vi "Database Change Manager UI.vi"(8 "error in (no error)":errorcluster, 10 "Old Cluster":refnum<k21>, 11 "VS Existing Frames":T1 {"Incoming"."Node Ref" format="%.0x"; "Outgoing"."Node Ref" format="%.0x"}) -> (0 "error out":errorcluster, 2 "Cancel Out":bool, 3 "Change":T5 {"Outgoing"."Frames to Update"."Node Ref" format="%.0x"; "Outgoing"."Frames to Delete" format="%.0x"; "Incoming"."Frames to Update"."Node Ref" format="%.0x"; "Incoming"."Frames to Delete" format="%.0x"})   [LabVIEW 2025, in "Protection and Counter Addon System Explorer.lvlib"]
uses:
  Protection and Counter Addon System Explorer.lvlib
  Types/CAN Update Results.ctl
  Types/VS Update List.ctl
  <vilib>/NI VeriStand/Custom Device API/Custom Device Item Ref.ctl
  Types/Base Frame Info_NoVS.ctl
  Types/Signal Attributes.ctl
  Types/CAN Filter Type.ctl
  Types/CAN Frame Update Results.ctl
  Types/Database Changes VS Existing Frames.ctl
  Types/Base Frame Info.ctl
  <vilib>/Utility/cursorutil.llb/Set Cursor (Icon Pict).vi
  <resource>/objmgr/xnet.rc
  <vilib>/NI VeriStand/Custom Device API/Custom Device API.lvlib
panel:
  in  "New Cluster":u16(ring)
  in  "New Database":refnum<k21>
  in  "Export":bool
  in  "Cancel":bool
  in  "Update":bool
  in  "Tree":string(tree)
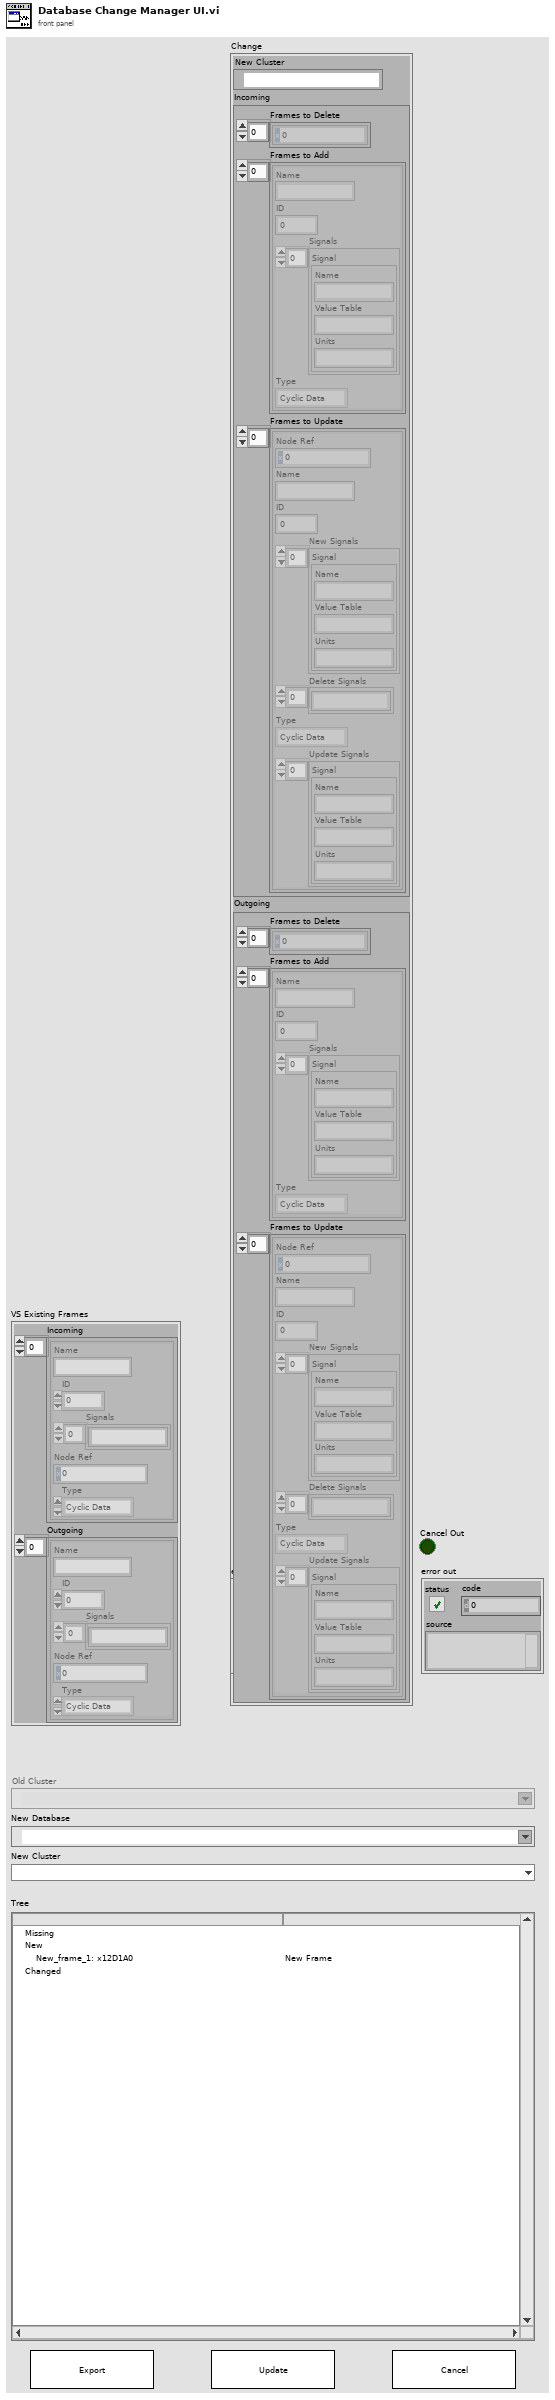
[diagram p1: front panel]
types:
  T1 = typedef "Protection and Counter Addon System Explorer.lvlib/Database Changes VS Existing Frames.ctl" = cluster{"Incoming":T2[], "Outgoing":T2[]}
  T2 = typedef "Protection and Counter Addon System Explorer.lvlib/Base Frame Info.ctl" = cluster{"Name":string, "ID":u32, "Signals":string[], "Node Ref":T3, "Type":T4}
  T3 = typedef "Custom Device API.lvlib/Custom Device Item Ref.ctl" = u64
  T4 = typedef "Protection and Counter Addon System Explorer.lvlib/CAN Filter Type.ctl" = enum16{"Cyclic Data", "Event Data", "Cyclic/Event", "All"}
  T5 = typedef "Protection and Counter Addon System Explorer.lvlib/CAN Update Results.ctl" = cluster{"New Cluster":refnum<k21>, "Incoming":T6, "Outgoing":T6}
  T6 = typedef "Protection and Counter Addon System Explorer.lvlib/VS Update List.ctl" = cluster{"Frames to Delete":T3[], "Frames to Add":T7[], "Frames to Update":T9[]}
  T7 = typedef "Protection and Counter Addon System Explorer.lvlib/Base Frame Info_NoVS.ctl" = cluster{"Name":string, "ID":u32, "Signals":T8[], "Type":T4}
  T8 = typedef "Protection and Counter Addon System Explorer.lvlib/Signal Attributes.ctl" = cluster{"Name":string, "Value Table":string, "Units":string}
  T9 = typedef "Protection and Counter Addon System Explorer.lvlib/CAN Frame Update Results.ctl" = cluster{"Node Ref":T3, "Name":string, "ID":u32, "New Signals":T8[], "Delete Signals":string[], "Type":T4, "Update Signals":T8[]}
  T10 = enum8{"Enabled", "Disabled", "Disabled and Grayed Out"}
  T11 = typedef "Protection and Counter Addon System Explorer.lvlib/Filtered XNET Changes.ctl" = cluster{"Incoming":T12, "Outgoing":T12}
  T12 = typedef "Protection and Counter Addon System Explorer.lvlib/Database Changes.ctl" = cluster{"New":T7[], "Missing":T2[], "Changed":T13[]}
  T13 = typedef "Protection and Counter Addon System Explorer.lvlib/Related CAN Frames.ctl" = cluster{"Old":T2, "Change":T14}
  T14 = typedef "Protection and Counter Addon System Explorer.lvlib/Related CAN Frames No VS.ctl" = cluster{"New":T7, "Old":T7}
  T15 = typedef "LVPoint32TypeDef.ctl" = cluster{"Horizontal":i32, "Vertical":i32}
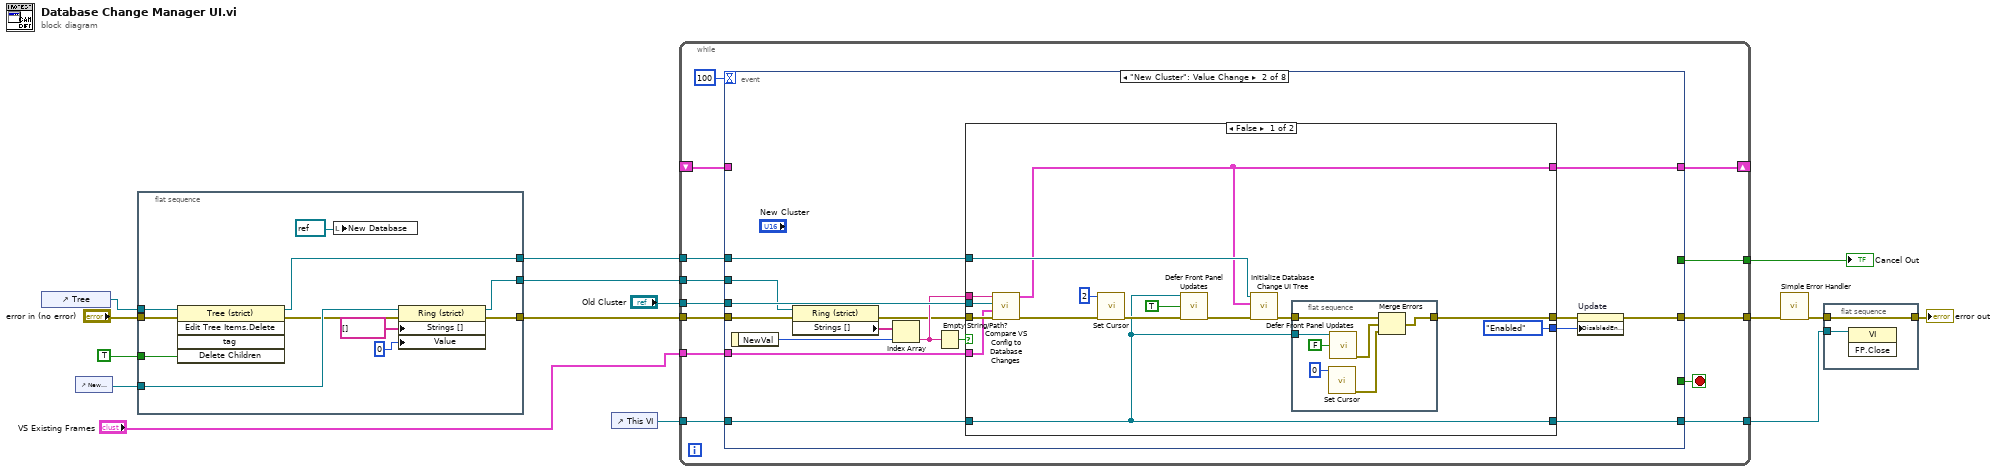
[diagram p0: block diagram]
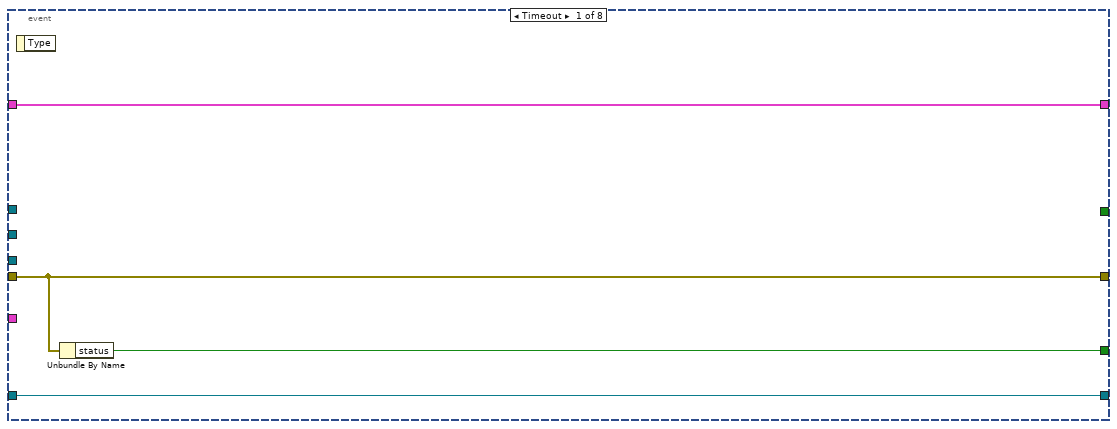
[diagram p2: hidden frame]
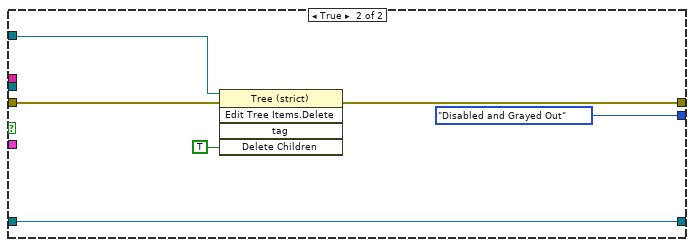
[diagram p3: hidden frame]
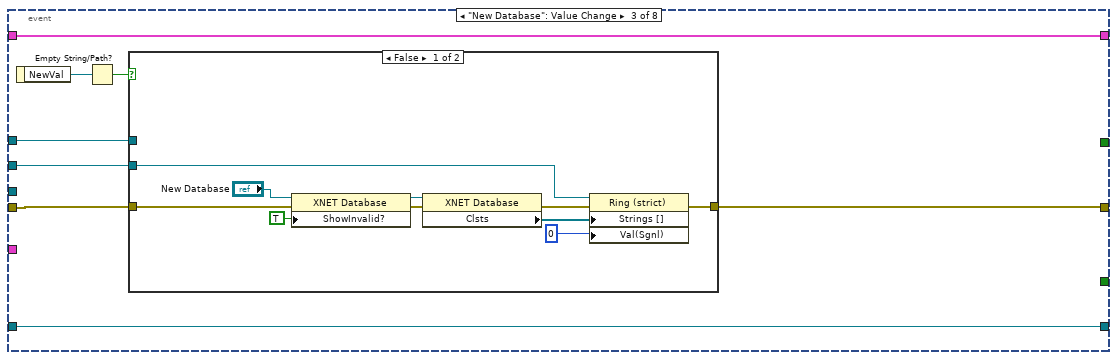
[diagram p4: hidden frame]
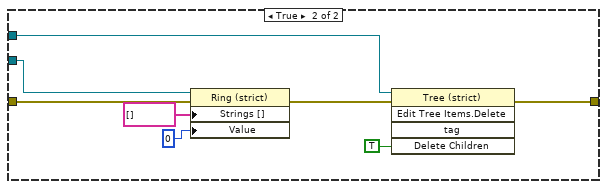
[diagram p5: hidden frame]
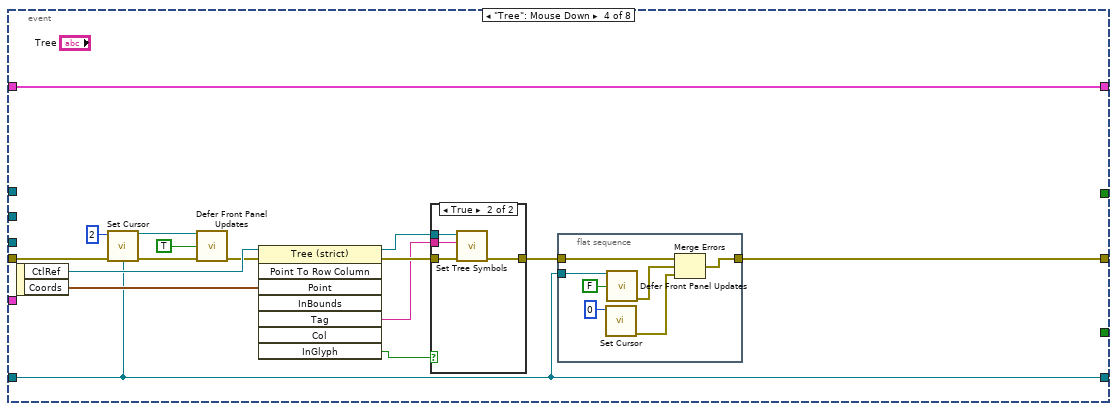
[diagram p6: hidden frame]
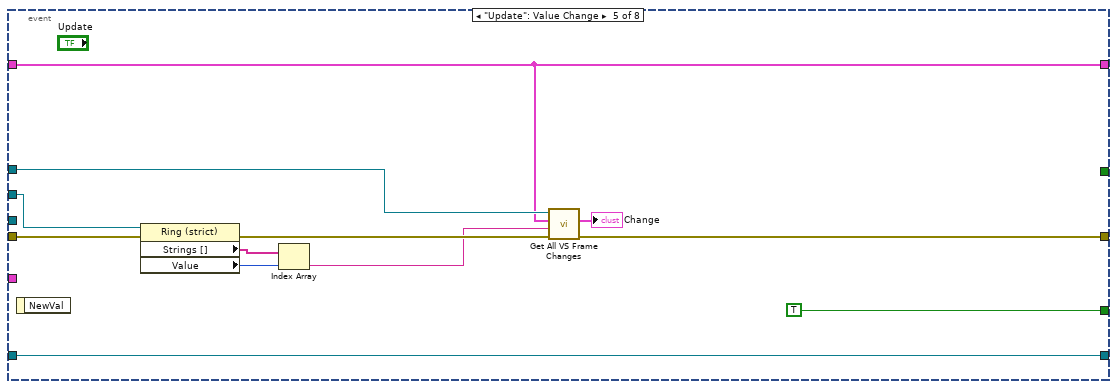
[diagram p8: hidden frame]
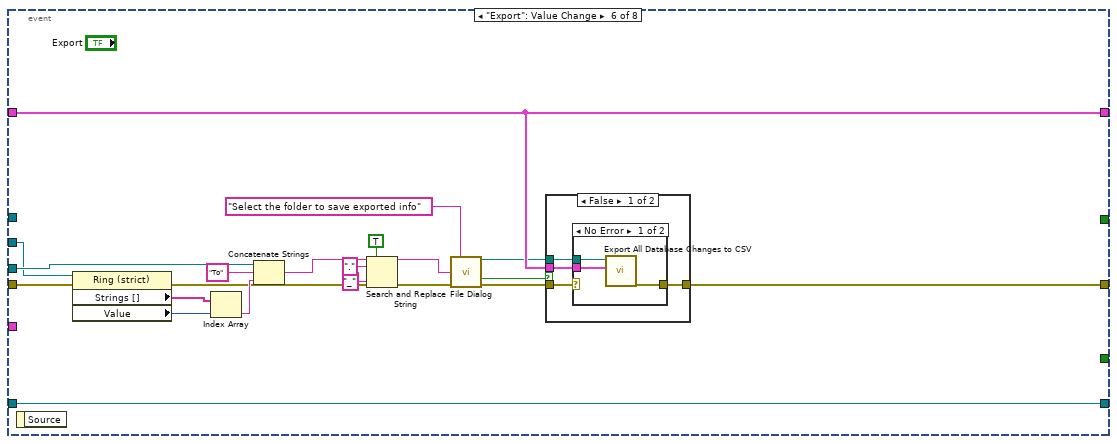
[diagram p9: hidden frame]
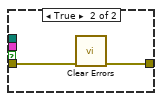
[diagram p11: hidden frame]
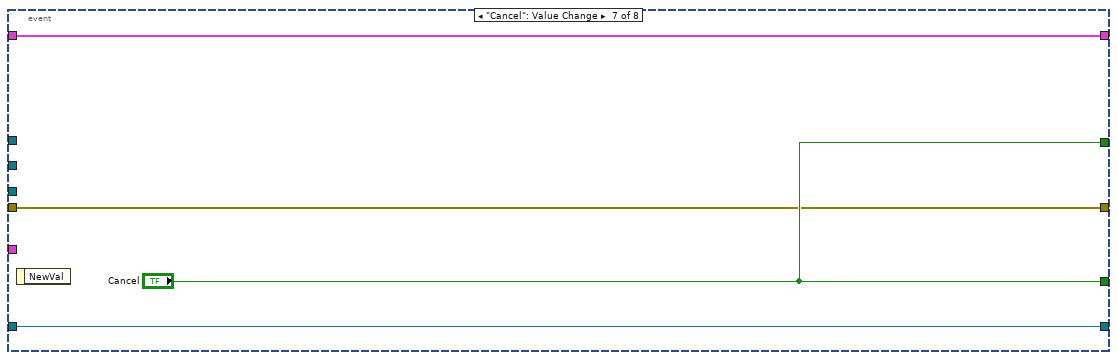
[diagram p12: hidden frame]
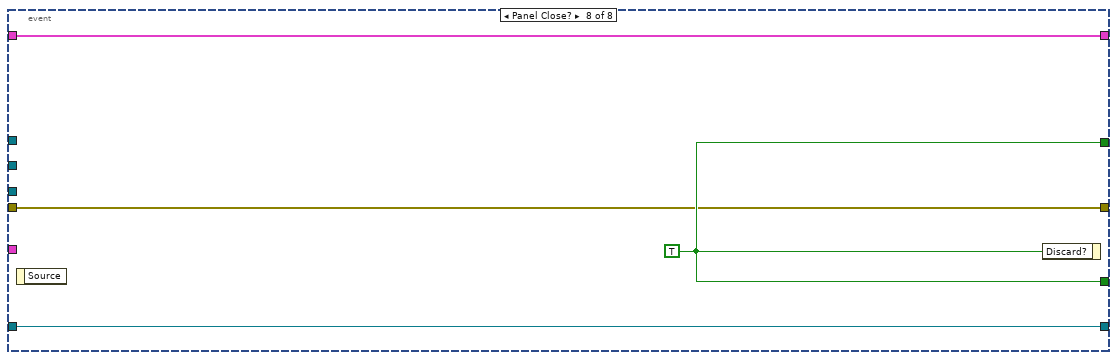
[diagram p13: hidden frame]
diagram:
  n1 = control-ref of="Tree"() -> (w7:refnum<vi>)
  n2 = control-ref of="New Cluster"() -> (w3:refnum<vi>)
  n3 = flat-sequence {
    tunnel: TRUE ("Delete Children?") -> [w26]
    tunnel: w7 -> [w25]
    tunnel: [w24] -> w6
    tunnel: "error in (no error)" -> [w23]
    tunnel: [w18] -> w4
    tunnel: w3 -> [w22]
    tunnel: [w17] -> w2
    frame #0 {
      n4 = invoke on="Invoke Node" class="Tree (strict)" method="Edit Tree Items.Delete"(reference=w25, error in=w23, "Delete Children"=w26) -> (reference out=w24:refnum<vi>, error out=w19:errorcluster)  [unwired: 2 in, 3 out]
      n5 = local write "New Database"(refnum<k21> refnum ("New Database")) -> ()
      n6 = property on="Property Node" class="Ring (strict)"(reference=w22, error in=w19, "Strings []"=string[] [], "Value"=u16 0) -> (reference out=w17:refnum<vi>, error out=w18:errorcluster)
    }
  }
  n7 = control-ref of="This VI"() -> (w9:refnum<vi>)
  n8 = while {
    tunnel: [w38] -> w14
    tunnel: [w37] -> w13
    tunnel: [w36] -> w12
    tunnel: "Old Cluster" -> [w34]
    tunnel: w6 -> [w33]
    tunnel: w9 -> [w32]
    tunnel: w4 -> [w31]
    shift-right: [w30] -> _
    shift-left: _ -> [w29]
    tunnel: "VS Existing Frames" -> [w28]
    tunnel: w2 -> [w27]
    stop <- w39 stop-if-true
    n9 = event shown="[1] \"New Cluster\": Value Change" {
      selector: _ -> [_ _ _ _ _ _ _ _]
      dyn-events: _ -> [_ _ _ _ _ _ _ _]
      timeout: 100 -> [_ _ _ _ _ _ _ _]
      tunnel: [w43 _ _ _ TRUE ("status") _ "Cancel" w191] -> w39
      tunnel: [w42 w52 w90 w120 w151 w153 w186 w190] -> w38
      tunnel: [w41 w55 w89 w116 w150 w173 w185 w189] -> w37
      tunnel: [_ _ _ _ _ _ "Cancel" w191] -> w36
      tunnel: w34 -> [_ w59 _ _ _ w168 _ _]
      tunnel: w33 -> [_ w58 w88 _ w149 _ _ _]
      tunnel: w32 -> [w41 w57 w89 w116 w150 w173 w185 w189]
      tunnel: w31 -> [w42 w45 w92 w115 w144 w163 w186 w190]
      tunnel: [w40 w56 w95 w114 w148 w172 w184 w188] -> w30
      tunnel: w29 -> [w40 _ w95 w114 w148 w172 w184 w188]
      tunnel: w28 -> [_ w50 _ _ _ _ _ _]
      tunnel: w27 -> [_ w44 w91 _ w146 w164 _ _]
      event Timeout {
        n10 = event-data() -> ()  [unwired: 1 in, 1 out]
        n11 = Unbundle By Name(w42) -> ("status"=w43:bool)
      }
      event "New Cluster": Value Change {
        n12 = event-data() -> ("NewVal"=w48:u16)  [unwired: 1 in]
        n13 = property class="Ring (strict)"(reference=w44, error in=w45) -> (error out=w46:errorcluster, "Strings []"=w49:string[])  [unwired: 1 out]
        n14 = Index Array(array=w49, index=w48) -> (element=w47:string)
        n15 = Empty String/Path?(string/path=w47) -> (empty?=w54:bool)
        n16 = case shown="False" w54 {
          tunnel: w59 -> [w71 _]
          tunnel: w47 -> [w70 _]
          tunnel: w58 -> [w69 w82]
          tunnel: w46 -> [w66 w83]
          tunnel: w57 -> [w63 w87]
          tunnel: [w64 w84] -> w53
          tunnel: [w60 _] -> w56
          tunnel: [w63 w87] -> w55
          tunnel: [T10."Enabled" ("Disabled") T10."Disabled and Grayed Out" ("Disabled")] -> w51
          tunnel: w50 -> [w61 _]
          frame False {
            n17 = call "Compare VS Config to Database Changes.vi"("error in (no error)"=w66, "VS Existing Frames"=w61, "Old Cluster"=w71, "New Cluster"=w70) -> ("error out"=w65:errorcluster, "VS Filtered Change List"=w60:T11)  [unwired: 6 in]
            n18 = call-poly <vilib>:"Set Cursor.vi"("error in (no error)"=w65, "icon"=u16 2) -> ("error out"=w72:errorcluster)  [unwired: 8 in, 1 out]
            n19 = call "Defer Front Panel Updates.vi"("This VI"=w63, "Defer Panel Updates"=TRUE, "error in (no error)"=w72) -> ("error out"=w73:errorcluster)  [unwired: 12 in]
            n20 = call "Initialize Database Change UI Tree.vi"("error in (no error)"=w73, "VS Filtered Change List"=w60, "TreeControl in"=w69) -> ("error out"=w74:errorcluster)  [unwired: 7 in, 1 out]
            n21 = flat-sequence {
              tunnel: [w80] -> w64
              tunnel: w74 -> [w79]
              tunnel: w63 -> [w77]
              frame #0 {
                n22 = call-poly <vilib>:"Set Cursor.vi"("icon"=u16 0) -> ("error out"=w75:errorcluster)  [unwired: 9 in, 1 out]
                n23 = call "Defer Front Panel Updates.vi"("This VI"=w77, "Defer Panel Updates"=FALSE) -> ("error out"=w78:errorcluster)  [unwired: 13 in]
                n24 = Merge Errors(w79, w78, w75) -> (w80:errorcluster)
              }
            }
          }
          frame True {
            n25 = invoke on="Invoke Node" class="Tree (strict)" method="Edit Tree Items.Delete"(reference=w82, error in=w83, "Delete Children"=TRUE ("Delete Children?")) -> (error out=w84:errorcluster)  [unwired: 2 in, 4 out]
          }
        }
        n26 = property on="Update" class="Bool"(error in=w53, "DisabledEnum"=w51) -> (error out=w52:errorcluster)  [unwired: 1 in, 1 out]
      }
      event "New Database": Value Change {
        n27 = event-data() -> ("NewVal"=w94:refnum<k21>)  [unwired: 1 in]
        n28 = Empty String/Path?(string/path=w94) -> (empty?=w93:bool)
        n29 = case shown="False" w93 {
          tunnel: w92 -> [w100 w106]
          tunnel: w91 -> [w98 w108]
          tunnel: [w96 w111] -> w90
          tunnel: w88 -> [_ w113]
          frame False {
            n30 = property class="XNET Database"(reference="New Database", error in=w100, "ShowInvalid?"=TRUE ("Show Invalid From Open?")) -> (reference out=w105:refnum<k21>, error out=w104:errorcluster)
            n31 = property class="XNET Database"(reference=w105, error in=w104) -> (error out=w97:errorcluster, "Clsts"=w101:refnum<k21>[])  [unwired: 1 out]
            n32 = property on="Property Node" class="Ring (strict)"(reference=w98, error in=w97, "Strings []"=w101, "Val(Sgnl)"=u16 0 ("Value (Signaling)")) -> (error out=w96:errorcluster)  [unwired: 1 out]
          }
          frame True {
            n33 = property on="Property Node" class="Ring (strict)"(reference=w108, error in=w106, "Strings []"=string[] [], "Value"=u16 0) -> (error out=w107:errorcluster)  [unwired: 1 out]
            n34 = invoke on="Invoke Node" class="Tree (strict)" method="Edit Tree Items.Delete"(reference=w113, error in=w107, "Delete Children"=TRUE ("Delete Children?")) -> (error out=w111:errorcluster)  [unwired: 2 in, 4 out]
          }
        }
      }
      event "Tree": Mouse Down {
        n35 = event-data() -> ("CtlRef"=w127:refnum<vi>, "Coords"=w128:T15)  [unwired: 1 in]
        n36 = call-poly <vilib>:"Set Cursor.vi"("error in (no error)"=w115, "icon"=u16 2) -> ("error out"=w118:errorcluster)  [unwired: 8 in, 1 out]
        n37 = call "Defer Front Panel Updates.vi"("This VI"=w116, "Defer Panel Updates"=TRUE, "error in (no error)"=w118) -> ("error out"=w117:errorcluster)  [unwired: 12 in]
        n38 = invoke on="Invoke Node" class="Tree (strict)" method="Point To Row Column"(reference=w127, error in=w117, "Point"=w128) -> (reference out=w125:refnum<vi>, error out=w126:errorcluster, "Tag"=w124:string, "InGlyph"=w123:bool)  [unwired: 5 in, 4 out]
        n39 = case shown="True" w123 {
          tunnel: w126 -> [w136 w140]
          tunnel: w125 -> [_ w139]
          tunnel: w124 -> [_ w138]
          tunnel: [w136 w137] -> w121
          frame False {
          }
          frame True {
            n40 = call "Set Tree Symbols.vi"("error in"=w140, "Tag"=w138, "CtlRef"=w139) -> ("error out"=w137:errorcluster)  [unwired: 8 in]
          }
        }
        n41 = flat-sequence {
          tunnel: [w132] -> w120
          tunnel: w121 -> [w133]
          tunnel: w116 -> [w129]
          frame #0 {
            n42 = call-poly <vilib>:"Set Cursor.vi"("icon"=u16 0) -> ("error out"=w134:errorcluster)  [unwired: 9 in, 1 out]
            n43 = call "Defer Front Panel Updates.vi"("This VI"=w129, "Defer Panel Updates"=FALSE) -> ("error out"=w130:errorcluster)  [unwired: 13 in]
            n44 = Merge Errors(w133, w130, w134) -> (w132:errorcluster)
          }
        }
      }
      event "Update": Value Change {
        n45 = event-data() -> ()  [unwired: 1 in, 1 out]
        n46 = property on="Property Node" class="Ring (strict)"(reference=w146, error in=w144) -> (error out=w145:errorcluster, "Strings []"=w143:string[], "Value"=w142:u16)  [unwired: 1 out]
        n47 = Index Array(array=w143, index=w142) -> (element=w141:string)
        n48 = call "Get All VS Frame Changes.vi"("error in (no error)"=w145, "New Cluster"=w141, "VS Filtered Change List"=w148, "TreeControl in"=w149) -> ("error out"=w151:errorcluster, "Change"=→"Change":T5)  [unwired: 5 in, 1 out]
      }
      event "Export": Value Change {
        n49 = event-data() -> ()  [unwired: 1 in, 1 out]
        n50 = property on="Property Node" class="Ring (strict)"(reference=w164, error in=w163) -> (error out=w159:errorcluster, "Strings []"=w162:string[], "Value"=w165:u16)  [unwired: 1 out]
        n51 = Index Array(array=w162, index=w165) -> (element=w161:string)
        n52 = Concatenate Strings(w168, "To" ("string"), w161) -> (w157:string)
        n53 = Search and Replace String(replace all?=TRUE ("replace all? (F)"), input string=w157, search string=".", replace string="_" ("replace string (\"\")"), error in=w159) -> (result string=w160:string, error out=w158:errorcluster)  [unwired: 3 in, 2 out]
        n54 = call "File Dialog"("prompt"="Select the folder to save exported info", "default name"=w160, "error in"=w158) -> ("selected path"=w171:path, "cancelled"=w170:bool, "error out"=w169:errorcluster)  [unwired: 9 in, 1 out]
        n55 = case shown="False" w170 {
          tunnel: w172 -> [w177 _]
          tunnel: w171 -> [w176 _]
          tunnel: w169 -> [w174 w183]
          tunnel: [w175 w182] -> w153
          frame False {
            n56 = case shown="No Error" w174 {
              selector: w174 -> [_ w181]
              tunnel: w177 -> [w180 _]
              tunnel: w176 -> [w179 _]
              tunnel: [w178 w181] -> w175
              frame No Error {
                n57 = call "Export All Database Changes to CSV.vi"("VS Filtered Change List"=w180, "Folder"=w179) -> ("error out"=w178:errorcluster)  [unwired: 9 in]
              }
              frame Error {
              }
            }
          }
          frame True {
            n58 = call <vilib>:"Clear Errors.vi"("error in (no error)"=w183) -> ("error out"=w182:errorcluster)  [unwired: 5 in, 1 out]
          }
        }
      }
      event "Cancel": Value Change {
        n59 = event-data() -> ()  [unwired: 1 in, 1 out]
      }
      event Panel Close? {
        w191 = TRUE ("Discard?")
        n60 = event-data() -> ()  [unwired: 1 in, 1 out]
        n61 = event-data("Discard?"=w191) -> ()  [unwired: 1 in, 1 out]
      }
    }
  }
  "Cancel Out" <- w12
  n62 = call <vilib>:"Simple Error Handler.vi"("error in (no error)"=w14) -> ("error out"=w15:errorcluster)  [unwired: 4 in, 4 out]
  n63 = flat-sequence {
    tunnel: [w193] -> w11
    tunnel: w15 -> [w193]
    tunnel: w13 -> [w192]
    frame #0 {
      n64 = invoke class="VI" method="FP.Close"(reference=w192) -> ()  [unwired: 2 in, 3 out]
    }
  }
  "error out" <- w11
